vi "PI_WAV_line_dyn.vi"(5 "Attach to wav":bool, 7 "Axis Identifier":string, 8 "Amplitude / [mu]":dbl, 9 "Startpos / [mu]":dbl, 10 "Pixel per scan":u16, 11 "Commandset in":string[](array[string])) -> (1 "Curve-Start-Pixel":i32, 2 "Num_Pix":u16, 3 "Commandset out":string[](array[string]))   [LabVIEW 2009]
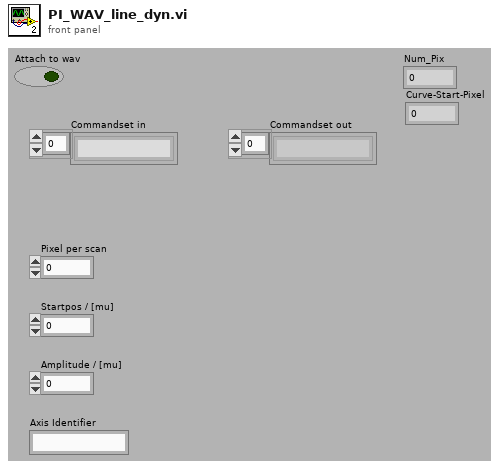
[diagram p1: front panel]
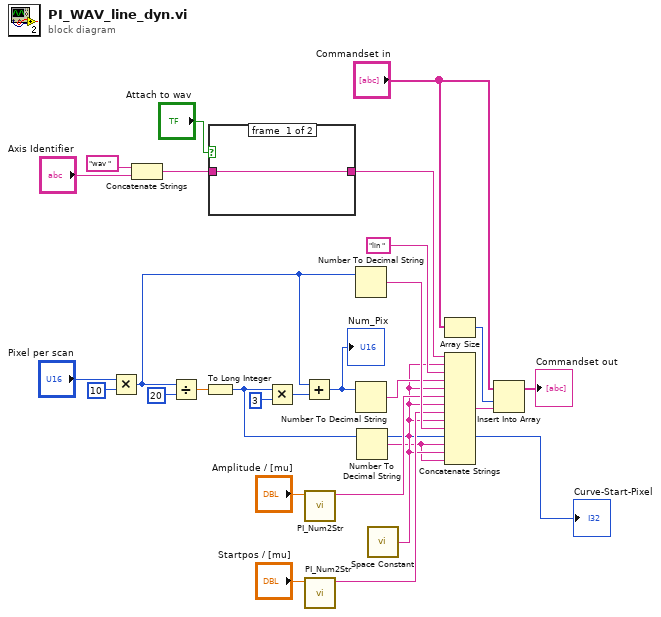
[diagram p0: block diagram]
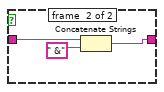
[diagram p2: hidden frame]
diagram:
  n1 = Multiply(x="Pixel per scan", y=u16 10) -> (x*y=w1:u16)
  n2 = Concatenate Strings("wav " ("new element/subarray"), "Axis Identifier") -> (w12:string)
  n3 = Divide(x=w1, y=u16 20) -> (x/y=w7:dbl)
  n4 = To Long Integer(number=w7) -> (32bit integer=w4:i32)
  "Curve-Start-Pixel" <- w4
  n5 = case shown="False" "Attach to wav" {
    tunnel: w12 -> [w28 w31]
    tunnel: [w28 w29] -> w11
    frame #0 {
    }
    frame #1 {
      n6 = Concatenate Strings(w31, " &" ("string")) -> (w29:string)
    }
  }
  n7 = Multiply(x=w4, y=3) -> (x*y=w5:i32)
  n8 = Add(x=w1, y=w5) -> (x+y=w19:i32)
  "Num_Pix" <- w19
  n9 = call "PI_Num2Str.vi"("x-Position"="Amplitude / [mu]") -> ("String"=w24:string)  [unwired: 10 out]
  n10 = call "PI_Num2Str.vi"("x-Position"="Startpos / [mu]") -> ("String"=w25:string)  [unwired: 10 out]
  n11 = Number To Decimal String(number=w1) -> (decimal integer string=w27:string)  [unwired: 1 out]
  n12 = Number To Decimal String(number=w19) -> (decimal integer string=w21:string)  [unwired: 1 out]
  n13 = Number To Decimal String(number=w4) -> (decimal integer string=w2:string)  [unwired: 1 out]
  n14 = call <vilib>:"Space Constant.vi"() -> ("String"=w3:string)
  n15 = Array Size(array="Commandset in") -> (size(s)=w15:i32)
  n16 = Concatenate Strings(w11, w3, "lin " ("string"), w21, w3, w24, w3, w25, w3, w27, w3, w2, w3, w2) -> (w22:string)
  n17 = Insert Into Array(array="Commandset in", index=w15, new element=w22) -> (→"Commandset out":string[])
